vi "Insert Parallel.vi"(8 "error in (no error)":errorcluster, 10 "Insert Parallel":T1, 11 "Test Executive Builder in":refnum<class "Test Executive Builder.lvclass">) -> (0 "error out":errorcluster, 3 "Test Executive Builder out":refnum<class "Test Executive Builder.lvclass">, 5 "Unique ID out":string)   [LabVIEW 2017, in "Test Executive Builder.lvclass"]
uses:
  Test Executive Builder.lvclass
  C:/Users/jonmc/Documents/Git/Test Executive Builder/Source/Test Executive Builder Model/Test Executive Builder Model/Test Executive Builder Model.lvclass
  C:/Users/jonmc/Documents/Git/Test Executive Builder/gpm_packages/@cs/mva-core/Source/IModel/IModel/IModel.lvclass
  Source/Application Dependencies/Insert Parallel.ctl
  Source/Test Executive Builder Model/Test Executive Builder Model/Test Executive Builder Model.lvclass/Test Executive Builder Model.ctl
  Test Executive Builder.lvclass/Test Executive Builder.ctl
  gpm_packages/@cs/mva-core/Source/IObserver/IObserver/IObserver.lvclass/IObserver.ctl
  gpm_packages/@cs/mva-core/Source/IModel/IModel/IModel.lvclass/IModel.ctl
  gpm_packages/@cs/mva-core/Source/IMediator/PublishRequest/PublishRequest.lvclass/PublishRequest.ctl
  gpm_packages/@cs/mva-core/Source/IMediator/IMediator Messages/Publish Msg/Publish Msg.lvclass/Publish Msg.ctl
  gpm_packages/@cs/actor-framework-messages/Source/RoundTripMessage/RoundTripMessage.lvclass/RoundTripMessage.ctl
  <vilib>/ActorFramework/Message Enqueuer/Message Enqueuer.lvclass/Message Enqueuer.ctl
  d5ddd591-8d14-4bb4-abf5-083b5114ca16.vi
  gpm_packages/@cs/mva-core/Source/IMediator/IMediator Messages/Publish Msg/Send Pre-Addressed Publish.vi
  gpm_packages/@cs/mva-core/Source/IObserver/IObserver/Read Unique ID.vi
  gpm_packages/@cs/mva-core/Source/IMediator/PublishRequest/Pack Publish Request.vi
  gpm_packages/@cs/actor-framework-messages/Source/RoundTripMessage/Return Round-Trip Message.vi
  <vilib>/ActorFramework/Message Enqueuer/Enqueue.vi
  gpm_packages/@cs/mva-core/Source/IModel/IModel/IModel.lvclass
  C:/Users/jonmc/Documents/Git/Test Executive Builder/gpm_packages/@cs/mva-core/Source/IObserver/IObserver/IObserver.lvclass
  gpm_packages/@cs/mva-core/Source/IMediator/IMediator Messages/Publish Msg/Publish Msg.lvclass
  C:/Users/jonmc/Documents/Git/Test Executive Builder/gpm_packages/@cs/actor-framework-messages/Source/RoundTripMessage/RoundTripMessage.lvclass
  gpm_packages/@cs/actor-framework-messages/Source/RoundTripMessage/RoundTripMessage.lvclass
  C:/Program Files (x86)/National Instruments/LabVIEW 2017/vi.lib/ActorFramework/Message/Message.lvclass
  <vilib>/Utility/error.llb/Error Cluster From Error Code.vi
  <vilib>/ActorFramework/Message Priority Queue/Priority Enqueue.vi
  Source/Test Executive Builder Model/Test Executive Builder Model/Test Executive Builder Model.lvclass
  gpm_packages/@cs/test-executive/Source/Test Executive/ITestExecutive/ITest Executive.lvclass
  gpm_packages/@cs/mva-core/Source/IMediator/PublishRequest/PublishRequest.lvclass
  Source/Test Executive Builder Dialogs/ITest Executive Builder Dialog/ITest Executive Builder Dialog.lvclass
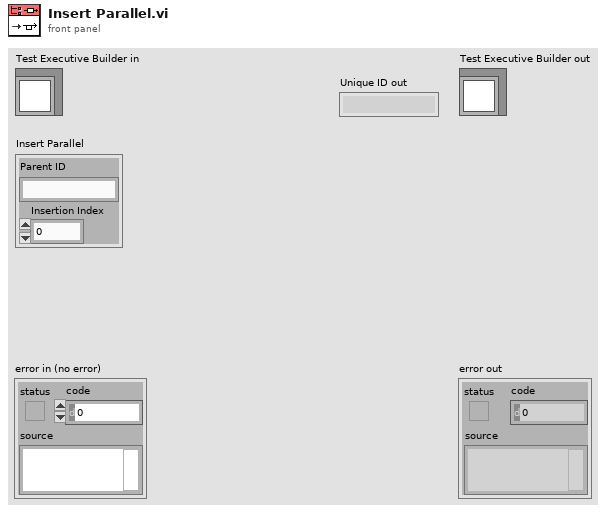
[diagram p1: front panel]
types:
  T1 = typedef "Insert Parallel.ctl" = cluster{"Parent ID":string, "Insertion Index":i32}
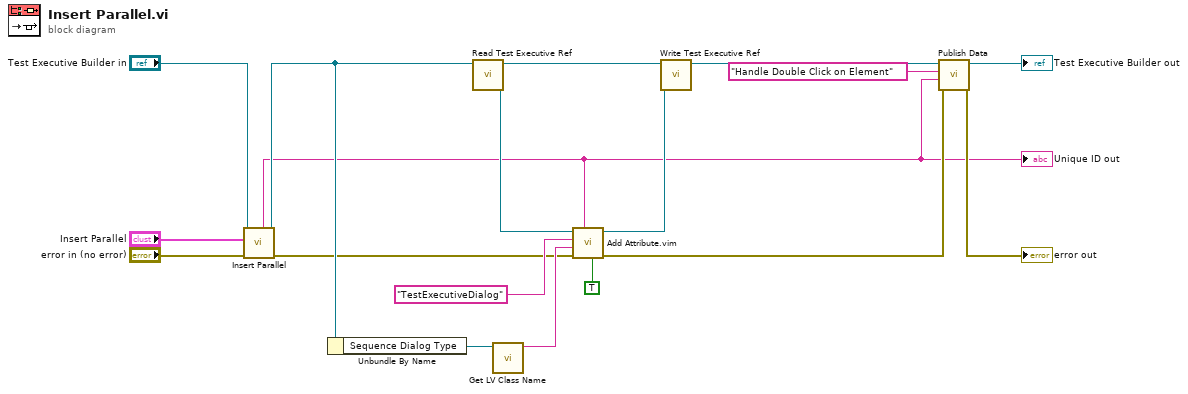
[diagram p0: block diagram]
diagram:
  n1 = call-parent "Insert Parallel.vi"("error in (no error)"="error in (no error)", "Insert Parallel"="Insert Parallel", "Test Executive Builder Model in"="Test Executive Builder in") -> ("error out"=w3:errorcluster, "Test Executive Builder Model out"=w5:refnum<class "Test Executive Builder.lvclass">, "Unique ID out"=w1:string)  [unwired: 6 in]
  "Unique ID out" <- w1
  n2 = Unbundle By Name(w5) -> ("Sequence Dialog Type"=w6:refnum<class "ITest Executive Builder Dialog.lvclass">)
  n3 = call "Read Test Executive Ref.vi"("Test Executive Builder Model in"=w5) -> ("Test Executive Ref"=w14:refnum<data-value>, "Test Executive Builder Model out"=w15:refnum<class "Test Executive Builder.lvclass">)  [unwired: 9 in]
  n4 = call <vilib>:"Get LV Class Name.vi"("object"=w6) -> ("class name"=w10:string)  [unwired: 9 in, 1 out]
  n5 = call "Add Attribute.vim"("Private?"=TRUE, "ID"=w1, "error in (no error)"=w3, "Attribute"=w10, "Attribute Name"="TestExecutiveDialog", "Test Executive Ref"=w14) -> ("error out"=w7:errorcluster, "Test Executive Ref out"=w13:refnum<data-value>)  [unwired: 2 in, 2 out]
  n6 = call "Write Test Executive Ref.vi"("Test Executive Ref"=w13, "Test Executive Builder Model in"=w15) -> ("Test Executive Builder Model out"=w8:refnum<class "Test Executive Builder.lvclass">)  [unwired: 9 in]
  n7 = call "Publish Data.vi"("error in (no error)"=w7, "Data to Publish"=w1, "Datum Name"="Handle Double Click on Element", "IModel in"=w8) -> ("error out"=→"error out":errorcluster, "IModel out"=→"Test Executive Builder out":refnum<class "Test Executive Builder.lvclass">)  [unwired: 6 in]
